vi "Proxy_Convert.vi"(11 "Data - P":i16[](array[numeric])) -> (2 "Data - P":dbl[](array[numeric]))   [LabVIEW 2019]
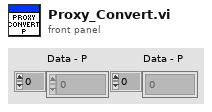
[diagram p1: front panel]
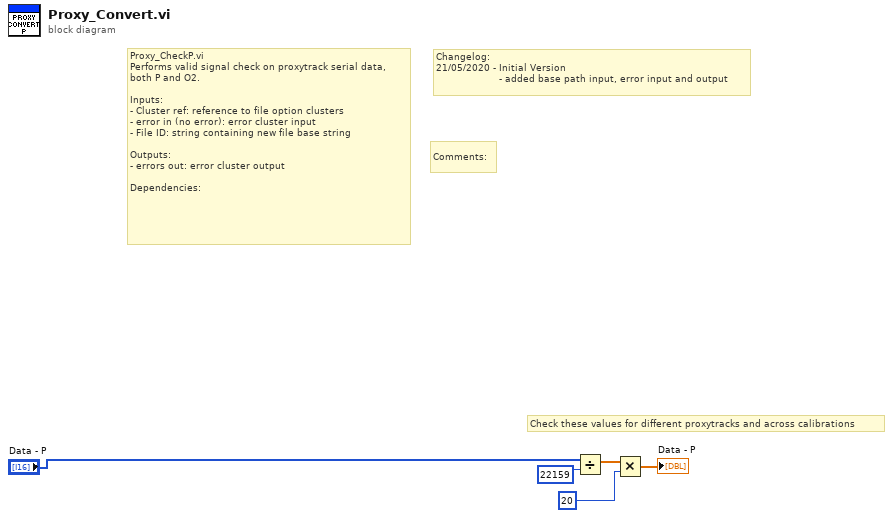
[diagram p0: block diagram]
diagram:
  # "Comments:"
  # "Changelog:\n21/05/2020 - Initial Version\n                     - added base path input, error input and output"
  # "Proxy_CheckP.vi\nPerforms valid signal check on proxytrack serial data,\nboth P and O2.\n\nInputs:\n- Cluster ref: reference to file option clusters\n- error in (no error): error cluster input\n- File ID: string containing new file base string\n\nOutputs:\n- errors out: error cluster output\n\nDependencies:"
  # "Check these values for different proxytracks and across calibrations"
  n1 = Divide(x="Data - P", y=22159) -> (x/y=w4:dbl[])
  n2 = Multiply(x=w4, y=20) -> (x*y=→"Data - P":dbl[])
